vi "Wave Generator(SubVI).vi"(0 "VISA Refnum in":refnum<visa-resource-name>, 1 "Channel (1:Channel 1)":i32(ring)=1 items=["Channel 1"=1, "Channel 2"=2], 2 "Fall (20 ns)":dbl=2e-08 format="%#.3g", 3 "Waveform Function (0: Sine) in":u16(ring) items=["Sine", "Square", "Ramp", "DC", "Pulse", "Arb"], 4 "Amplitude (1.0 Vpp)":dbl=1.0 format="%#.3f", 5 "Frequency (1000 Hz)":dbl=1000.0 format="%#.6g", 6 "DC Offset (0.00 V) in":dbl, 8 "Enable Output (T: Enable)":bool=TRUE, 9 "Delay (0.00 s)":dbl min=-1000000.0 max=1000000.0, 10 "Filename":string, 11 "Rise (20 ns)":dbl=2e-08 format="%#.3g", 12 "Duty (20%)":dbl=20.0 min=0.0001 max=100.0 format="%.4g", 13 "True To \ngenerate\n pulse":bool, 14 "format string":string, 15 "Phase (0.0 degrees)":dbl=0.002 min=-360.0 max=360.0 format="%#.1g", 16 "File Directory":path) -> (18 "Output Directory":path, 20 "VISA Refnum out":refnum<visa-resource-name>, 21 "Output Filename":path, 22 "error out 2":errorcluster, 27 "error out":errorcluster)   [LabVIEW 2018]
uses:
  <instrlib>/Siglent SDG X Series/Siglent SDG X Series.lvlib
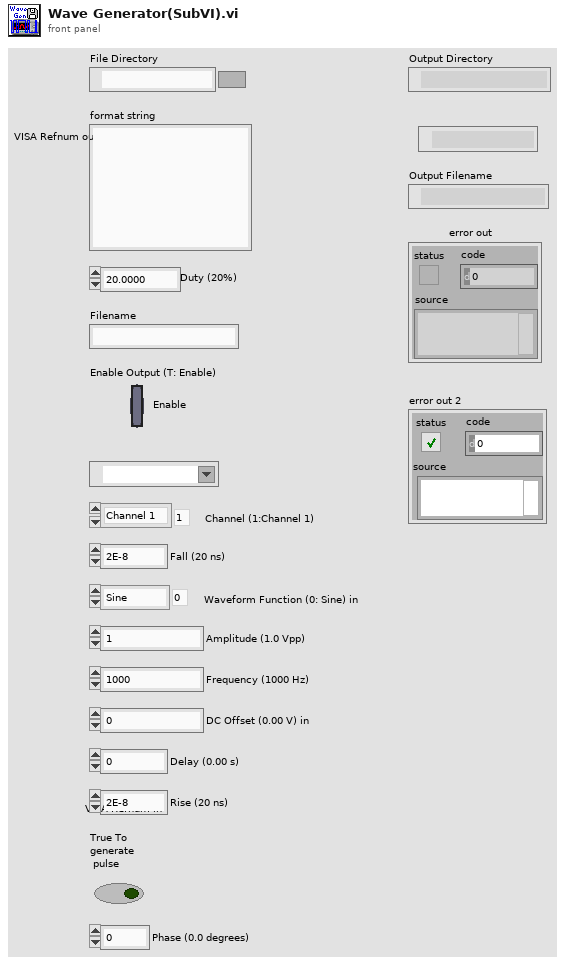
[diagram p1: front panel]
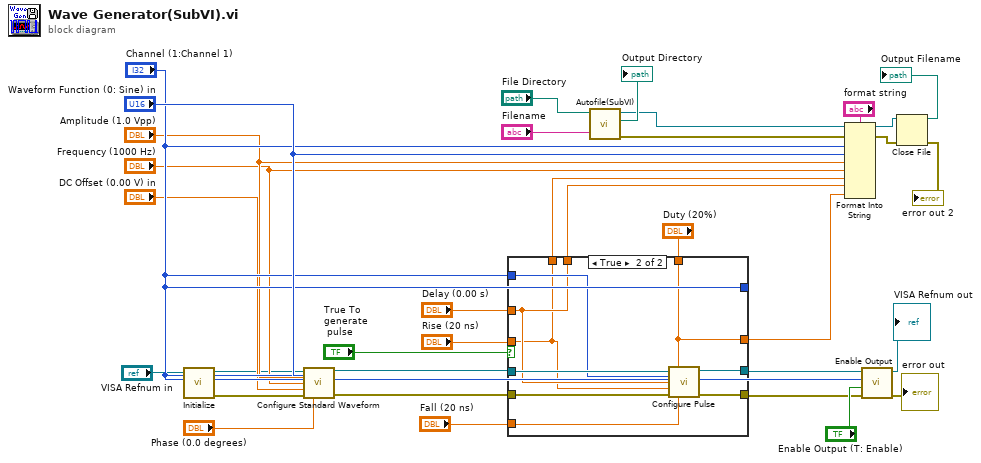
[diagram p0: block diagram]
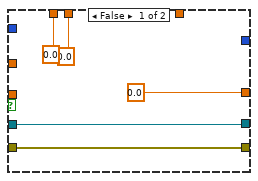
[diagram p2: hidden frame]
diagram:
  n1 = call <instrlib>:"Initialize.vi"("VISA resource name"="VISA Refnum in") -> ("error out"=w6:errorcluster, "VISA resource name out"=w5:refnum<visa-resource-name>)  [unwired: 9 in]
  n2 = call <instrlib>:"Configure Standard Waveform.vi"("VISA resource name"=w5, "Waveform Function (0: Sine)"="Waveform Function (0: Sine) in", "Channel (1:Channel 1)"="Channel (1:Channel 1)", "Amplitude (1.0 Vpp)"="Amplitude (1.0 Vpp)", "Frequency (1000 Hz)"="Frequency (1000 Hz)", "DC Offset (0.00 V)"="DC Offset (0.00 V) in", "error in (no error)"=w6, "Phase (0.0 degrees)"="Phase (0.0 degrees)") -> ("VISA resource name out"=w10:refnum<visa-resource-name>, "error out"=w7:errorcluster)  [unwired: 6 in]
  n3 = case shown="True" "True To \ngenerate\n pulse" {
    tunnel: [w39 w48] -> w1
    tunnel: [w38 w47] -> w2
    tunnel: w10 -> [w39 w46]
    tunnel: w7 -> [w38 w45]
    tunnel: "Channel (1:Channel 1)" -> [_ w44]
    tunnel: "Channel (1:Channel 1)" -> [_ _]
    tunnel: [0.0 ("Duty (20%)") w40] -> w14
    tunnel: [0.0 ("Rise (20 ns)") w41] -> w22
    tunnel: [0.0 ("Delay (0.00 s)") w42] -> w23
    tunnel: "Fall (20 ns)" -> [_ w43]
    tunnel: "Delay (0.00 s)" -> [_ w42]
    tunnel: "Rise (20 ns)" -> [_ w41]
    tunnel: "Duty (20%)" -> [_ w40]
    frame False {
    }
    frame True {
      n4 = call <instrlib>:"Configure Pulse.vi"("VISA resource name"=w46, "Duty (20%)"=w40, "Channel (1:Channel 1)"=w44, "Delay (0.00 s)"=w42, "Rise (20 ns)"=w41, "error in (no error)"=w45, "Fall (20 ns)"=w43) -> ("VISA resource name out"=w48:refnum<visa-resource-name>, "error out"=w47:errorcluster)  [unwired: 7 in]
    }
  }
  n5 = call "Autofile(SubVI).vi"("Filename"="Filename", "File Directory"="File Directory") -> ("error out"=w27:errorcluster, "Output Directory"=→"Output Directory":path, "Byte Stream File out"=w26:refnum<file>)  [unwired: 7 in]
  n6 = Format Into String(format string="format string", initial string=w26, error in=w27, "Channel (1:Channel 1)", "Waveform Function (0: Sine) in", "Amplitude (1.0 Vpp)", "Frequency (1000 Hz)", w22, w23, w14) -> (resulting string=w15:refnum<file>, error out=w18:errorcluster)
  n7 = call <instrlib>:"Enable Output.vi"("error in (no error)"=w2, "Enable Output (T: Enable)"="Enable Output (T: Enable)", "Channel (1:Channel 1)"="Channel (1:Channel 1)", "VISA resource name"=w1) -> ("error out"=→"error out":errorcluster, "VISA resource name out"=→"VISA Refnum out":refnum<visa-resource-name>)  [unwired: 6 in]
  n8 = Close File(refnum=w15, error in=w18) -> (path=→"Output Filename":path, error out=→"error out 2":errorcluster)
